vi "CetoniPump_Init.vi"(0 "object in":refnum<class "CetoniPump.lvclass">, 2 "Device Configuration Path":string="C:\\Users\\Public\\Documents\\QmixElements\\Projects\\default_project\\Configurations\\sinle", 5 "error in (no error)":errorcluster) -> (14 "object out":refnum<class "CetoniPump.lvclass">, 19 "error out":errorcluster)   [LabVIEW 2024, in "CetoniPump.lvclass"]
uses:
  CetoniPump.lvclass
  Users/Lab user/AppData/Local/CETONI_SDK/lib/labview/labbCAN_Bus_API/SiUnitPrefix.ctl
  Users/Lab user/AppData/Local/CETONI_SDK/lib/labview/labbCAN_Pump_API/VolumeUnits.ctl
  Users/Lab user/AppData/Local/CETONI_SDK/lib/labview/labbCAN_Bus_API/TimeUnits.ctl
  CetoniPump.lvclass/CetoniPump.ctl
  Users/Lab user/AppData/Local/CETONI_SDK/lib/labview/labbCAN_Bus_API/labbCAN_Bus_API.lvlib
  Users/Lab user/AppData/Local/CETONI_SDK/lib/labview/labbCAN_Pump_API/labbCAN_Pump_API.lvlib
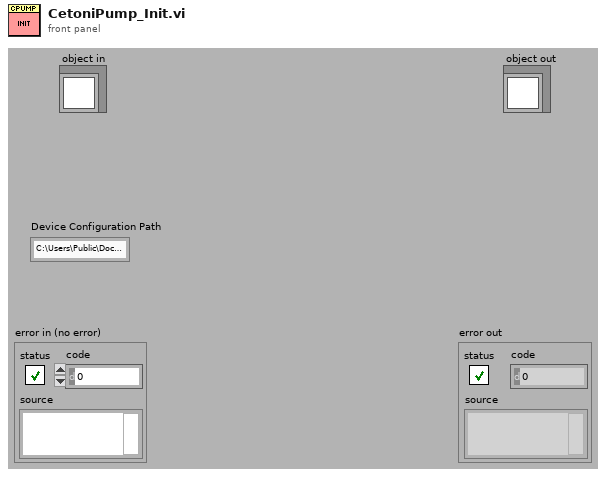
[diagram p1: front panel]
types:
  T1 = typedef "labbCAN_Bus_API.lvlib/TimeUnits.ctl" = i32
  T2 = typedef "labbCAN_Pump_API.lvlib/VolumeUnits.ctl" = i32
  T3 = typedef "labbCAN_Bus_API.lvlib/SiUnitPrefix.ctl" = i32
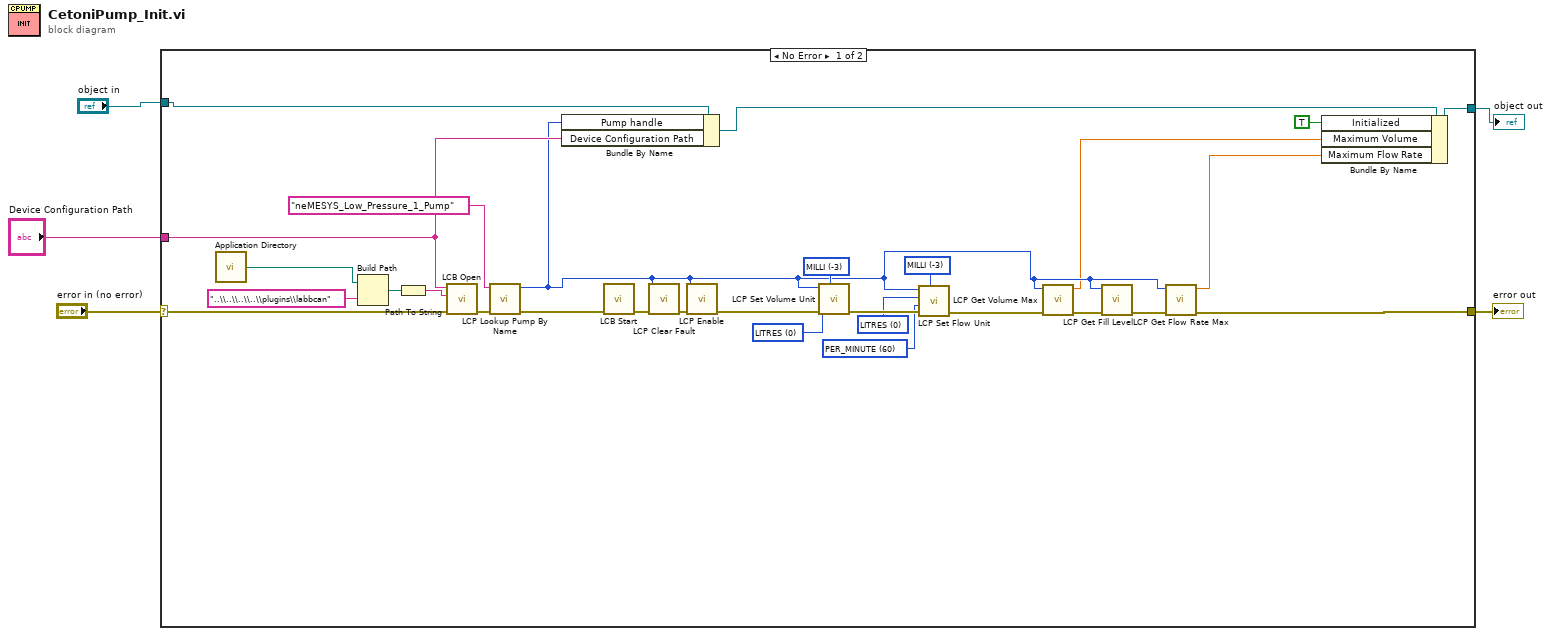
[diagram p0: block diagram]
diagram:
  n1 = case shown="No Error" "error in (no error)" {
    selector: "error in (no error)" -> [w24 w35]
    tunnel: "object in" -> [w34 w36]
    tunnel: [w11 w36] -> w4
    tunnel: [w7 w35] -> w2
    tunnel: "Device Configuration Path" -> [w23 _]
    frame No Error {
      w17 = T1 60 items=["PER_SECOND"=1, "PER_MINUTE"=60, "PER_HOUR"=3600] ("TimeUnit")
      w18 = T2 0 items=["LITRES"] ("VolumeUnit")
      w19 = T2 0 items=["LITRES"] ("Volume Unit")
      w20 = T3 -3 items=["UNIT"=0, "DECI"=-1, "CENTI"=-2, "MILLI"=-3, "MICRO"=-6] ("Prefix")
      w22 = T3 -3 items=["UNIT"=0, "DECI"=-1, "CENTI"=-2, "MILLI"=-3, "MICRO"=-6] ("Prefix")
      n2 = call <vilib>:"Application Directory.vi"() -> ("Application Directory"=w33:path)
      n3 = Build Path(base path=w33, name or relative path="..\\..\\..\\..\\plugins\\labbcan" ("Name oder relativer Pfad")) -> (appended path=w30:path)
      n4 = Path To String(path=w30) -> (string=w29:string)
      n5 = call "LCB Open.vi"("error in (no error)"=w24, "PluginSearchPath"=w29, "Device Configuration Path"=w23) -> ("error out"=w32:errorcluster)  [unwired: 8 in]
      n6 = call "LCP Lookup Pump By Name.vi"("error in (no error)"=w32, "Pump Name"="neMESYS_Low_Pressure_1_Pump" ("pAxisName")) -> ("error out"=w28:errorcluster, "Pump handle"=w13:i64)  [unwired: 8 in]
      n7 = Bundle By Name(cluster=w34, "Pump handle"=w13, "Device Configuration Path"=w23) -> (w12:refnum<class "CetoniPump.lvclass">)
      n8 = call "LCB Start.vi"("error in (no error)"=w28) -> ("error out"=w27:errorcluster)  [unwired: 10 in]
      n9 = call "LCP Clear Fault.vi"("error in (no error)"=w27, "Pump Handle"=w13) -> ("error out"=w26:errorcluster)  [unwired: 9 in]
      n10 = call "LCP Enable.vi"("error in (no error)"=w26, "Pump Handle"=w13) -> ("error out"=w16:errorcluster)  [unwired: 9 in]
      n11 = call "LCP Set Volume Unit.vi"("Prefix"=w22, "error in (no error)"=w16, "Volume Unit"=w19, "Pump Handle"=w13) -> ("error out"=w21:errorcluster)  [unwired: 7 in]
      n12 = call "LCP Set Flow Unit.vi"("Prefix"=w20, "error in (no error)"=w21, "TimeUnit"=w17, "VolumeUnit"=w18, "Pump Handle"=w13) -> ("error out"=w8:errorcluster)  [unwired: 6 in]
      n13 = call "LCP Get Volume Max.vi"("error in (no error)"=w8, "Pump Handle"=w13) -> ("error out"=w15:errorcluster, "Maximum Volume"=w10:dbl)  [unwired: 8 in]
      n14 = call "LCP Get Fill Level.vi"("error in (no error)"=w15, "Pump Handle"=w13) -> ("error out"=w14:errorcluster)  [unwired: 8 in, 1 out]
      n15 = call "LCP Get Flow Rate Max.vi"("error in (no error)"=w14, "Pump Handle"=w13) -> ("error out"=w7:errorcluster, "Maximum Flow Rate"=w9:dbl)  [unwired: 8 in]
      n16 = Bundle By Name(cluster=w12, "Initialized"=TRUE, "Maximum Volume"=w10, "Maximum Flow Rate"=w9) -> (w11:refnum<class "CetoniPump.lvclass">)
    }
    frame Error {
    }
  }
  "object out" <- w4
  "error out" <- w2
